vi "Rectangle Apply Inkscape Ratio.vi"(1 "rects in":T2(array[cluster])) -> (0 "rects out":T2(array[cluster]))   [LabVIEW 2016]
uses:
  <vilib>/Analysis/Matrix/Datatypes/RealMatrix.ctl
  Global Variables.vi
  <vilib>/Analysis/Matrix/NI_Matrix.lvlib
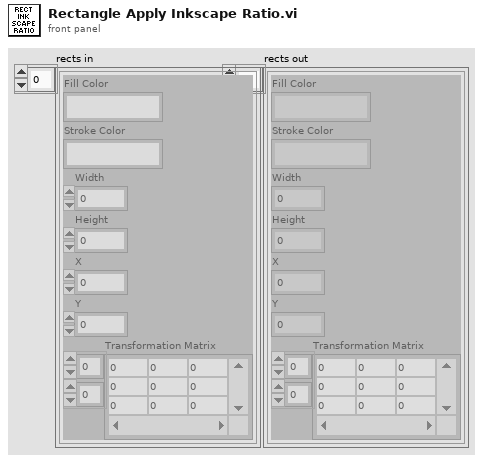
[diagram p1: front panel]
types:
  T1 = typedef "NI_Matrix.lvlib/RealMatrix.ctl" = dbl[][]
  T2 = cluster{"Fill Color":string, "Stroke Color":string, "Width":dbl, "Height":dbl, "X":dbl, "Y":dbl, "Transformation Matrix":T1}[]
  T3 = cluster{"Fill Color":string, "Stroke Color":string, "Width":dbl, "Height":dbl, "X":dbl, "Y":dbl, "Transformation Matrix":T1}
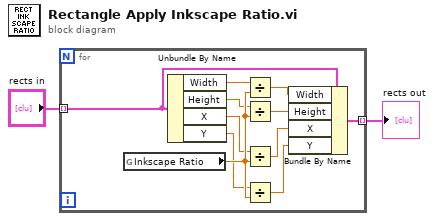
[diagram p0: block diagram]
diagram:
  n1 = for {
    tunnel: "rects in" -> [w4] mode=indexing
    tunnel: [w3] -> w2 mode=indexing
    n2 = global read "Global Variables.vi" "Inkscape Ratio"() -> (w13:dbl)
    n3 = Unbundle By Name(w4) -> ("Width"=w12:dbl, "Height"=w11:dbl, "X"=w10:dbl, "Y"=w9:dbl)
    n4 = Divide(x=w12, y=w13) -> (x/y=w8:dbl)
    n5 = Divide(x=w11, y=w13) -> (x/y=w7:dbl)
    n6 = Divide(x=w10, y=w13) -> (x/y=w6:dbl)
    n7 = Divide(x=w9, y=w13) -> (x/y=w5:dbl)
    n8 = Bundle By Name(cluster=w4, "Width"=w8, "Height"=w7, "X"=w6, "Y"=w5) -> (w3:T3)
  }
  "rects out" <- w2
